vi "Convert 2D image to RAW FPGA stream.vi"(8 "error in":errorcluster, 10 "image data":T1={"image type"=0, "image depth"=24, "image"=array[230400 elements], "mask"=[], "colors"=[], "Rectangle"={"left"=0, "top"=0, "right"=320, "bottom"=240}}, 11 "file path (use dialog)":path=path "\\\\vmware-host\\Shared Folders/Downloads/pug.bin") -> (0 "error out":errorcluster, 3 "data":u16[](array[numeric]) format="%.0x")   [LabVIEW 2019]
uses:
  <vilib>/picture/picture.llb/imagedata.ctl
  <userlib>/_OpenG.lib/file/file.llb/File Exists - Scalar__ogtk.vi
panel:
  out "exists":bool
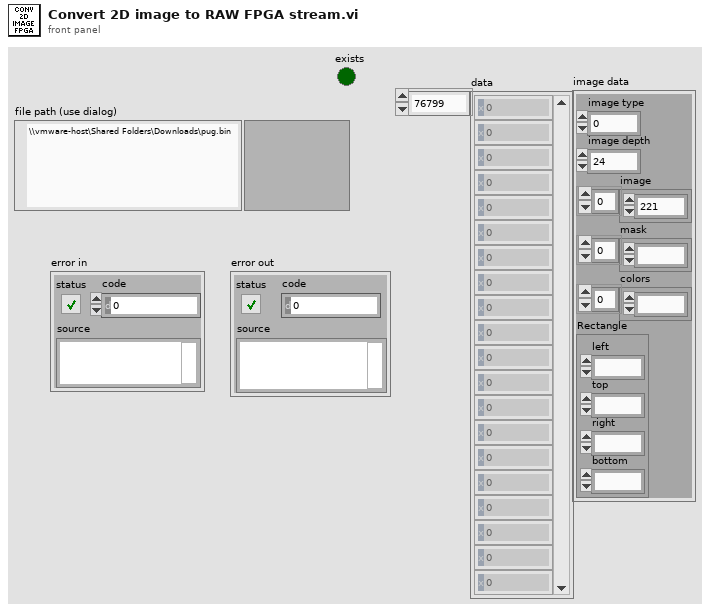
[diagram p1: front panel]
types:
  T1 = typedef "imagedata.ctl" = cluster{"image type":i32, "image depth":i32, "image":u8[], "mask":u8[], "colors":u32[], "Rectangle":cluster{"left":i16, "top":i16, "right":i16, "bottom":i16}}
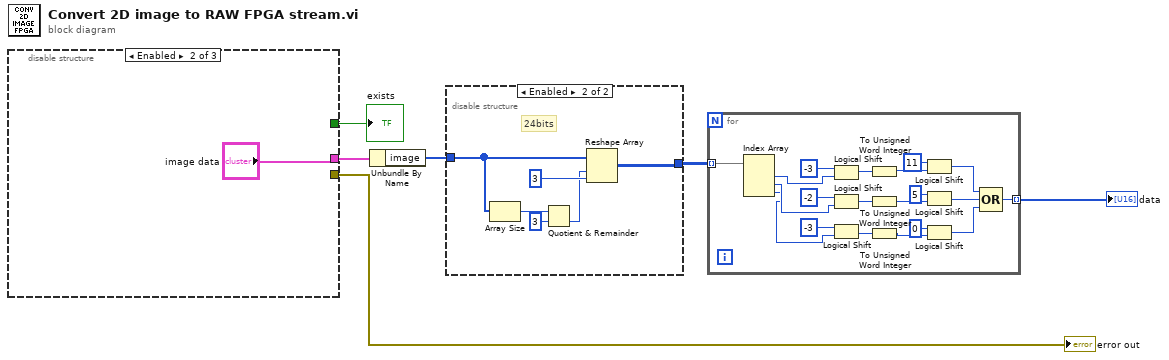
[diagram p0: block diagram]
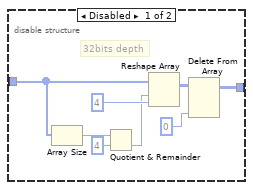
[diagram p2: hidden frame]
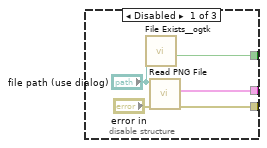
[diagram p3: hidden frame]
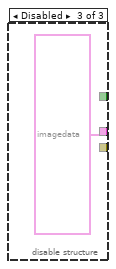
[diagram p4: hidden frame]
diagram:
  n1 = disable-structure shown="Enabled" {
    disable-tunnel: [w10 _ _] -> w3
    disable-tunnel: [w8 _ _] -> w2
    disable-tunnel: [w7 "image data" T1 {"image type"=0, "image depth"=24, "image"=array[230400 elements], "mask"=[], "colors"=[], "Rectangle"={"left"=0, "top"=0, "right"=320, "bottom"=240}} ("image data")] -> w1
    frame Disabled {
      n2 = call-poly <userlib>:"File Exists__ogtk.vi"("file path"="file path (use dialog)") -> ("exists"=w8:bool)  [unwired: 6 in, 1 out]
      n3 = call <vilib>:"Read PNG File.vi"("error in (no error)"="error in", "path to PNG file"="file path (use dialog)") -> ("error out"=w10:errorcluster, "image data"=w7:T1)  [unwired: 7 in, 1 out]
    }
    frame Enabled {
    }
    frame Disabled {
    }
  }
  "error out" <- w3
  "exists" <- w2
  n4 = Unbundle By Name(w1) -> ("image"=w6:u8[])
  n5 = disable-structure shown="Enabled" {
    disable-tunnel: w6 -> [w15 w23]
    disable-tunnel: [w14 w22] -> w5
    frame Disabled {
      # "32bits depth"
      n6 = Array Size(array=w15) -> (size(s)=w21:i32)
      n7 = Quotient & Remainder(x=w21, y=4) -> (floor(x/y)=w17:i32)  [unwired: 1 out]
      n8 = Reshape Array(w15, w17, 4 ("dimension size")) -> (w19:u8[][])
      n9 = Delete From Array(array=w19, index (col)=0 ("dimension size")) -> (array with subset deleted=w14:u8[][])  [unwired: 2 in, 1 out]
    }
    frame Enabled {
      # "24bits"
      n10 = Array Size(array=w23) -> (size(s)=w27:i32)
      n11 = Quotient & Remainder(x=w27, y=3) -> (floor(x/y)=w24:i32)  [unwired: 1 out]
      n12 = Reshape Array(w23, w24, 3 ("dimension size")) -> (w22:u8[][])
    }
  }
  n13 = for {
    tunnel: w5 -> [w47] mode=indexing
    tunnel: [w31] -> w4 mode=indexing
    n14 = Index Array(array=w47) -> (element #1=w30:u8, element #2=w29:u8, element #3=w28:u8)  [unwired: 3 in]
    n15 = Logical Shift(y=i16 -3, x=w30) -> (x << y=w43:u8)
    n16 = Logical Shift(y=i16 -2, x=w29) -> (x << y=w42:u8)
    n17 = Logical Shift(y=i16 -3, x=w28) -> (x << y=w41:u8)
    n18 = To Unsigned Word Integer(number=w43) -> (unsigned 16bit integer=w40:u16)
    n19 = To Unsigned Word Integer(number=w42) -> (unsigned 16bit integer=w37:u16)
    n20 = To Unsigned Word Integer(number=w41) -> (unsigned 16bit integer=w35:u16)
    n21 = Logical Shift(y=i16 11, x=w40) -> (x << y=w34:u16)
    n22 = Logical Shift(y=i16 5, x=w37) -> (x << y=w33:u16)
    n23 = Logical Shift(y=i16 0, x=w35) -> (x << y=w32:u16)
    n24 = Compound Arithmetic op=OR(w34, w33, w32) -> (w31:u16)
  }
  "data" <- w4
